vi "Response to Client.vi"(8 "error in (no error)":errorcluster, 9 "Context":variant, 10 "Message":variant, 11 "Communications in":refnum<class "Communications.lvclass">) -> (0 "error out":errorcluster, 1 "Context out":variant, 3 "Communications out":refnum<class "Communications.lvclass">)   [LabVIEW 2016, in "Communications.lvclass"]
uses:
  Communications.lvclass
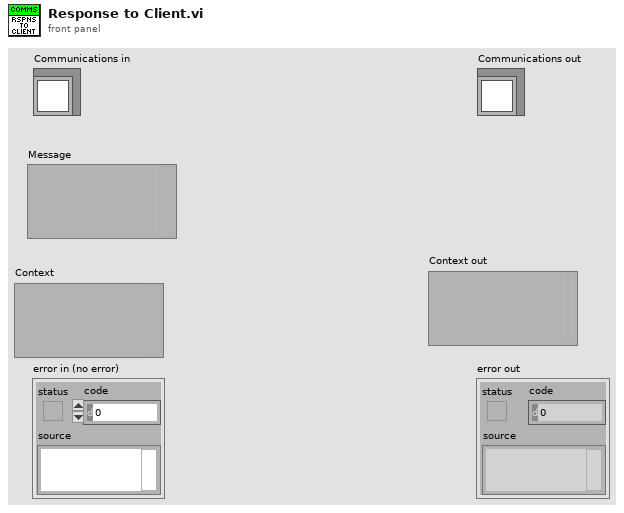
[diagram p1: front panel]
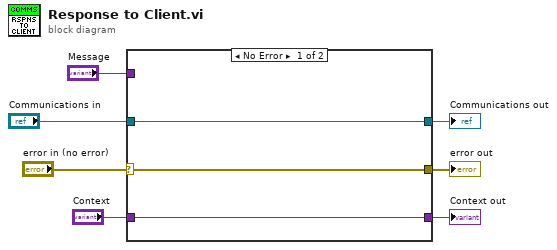
[diagram p0: block diagram]
diagram:
  n1 = case shown="No Error" "error in (no error)" {
    selector: "error in (no error)" -> [w9 w13]
    tunnel: [w9 w13] -> w6
    tunnel: [w10 w12] -> w4
    tunnel: "Communications in" -> [w10 w12]
    tunnel: "Context" -> [w8 w11]
    tunnel: [w8 w11] -> w2
    tunnel: "Message" -> [_ _]
    frame No Error {
    }
    frame Error {
    }
  }
  "error out" <- w6
  "Communications out" <- w4
  "Context out" <- w2
